vi "Recent History Buffer (Array(DBL)).vi"(8 "number of elements [init or read] (100)":i32=100, 9 "new element [write]":dbl format="%0.2f", 10 "mode [init:0;write:1;read:2]":enum16{"initialize", "write", "read"}(ring)) -> (1 "number to date":u32, 2 "requested elements [read]":dbl[](array[numeric]) format="%0.2f", 3 "buffer full?":bool)   [LabVIEW 2009]
doc: "This history buffer saves an internal 1D array of the most recent N values that it receives, where N is the number of elements specified when the buffer is initialized. \n\nThere are three modes to access this buffer - init, write, and read. You must first call the VI in init mode to set the buffer size. In write mode, each call writes a new element to the buffer, overwriting the oldest element if the buffer is full. In read mode, each call returns the lesser of the requested number of elements or the number currently stored in the buffer; element 0 is the oldest of the requested elements.\n\nSince this VI behaves like a global variable, it is called a \"functional global\". Search the LabVIEW Help for \"functional global\" for more information on the reasons you might use a functional global instead of a standard global variable."
panel:
  # "Press Ctrl-H for more information."
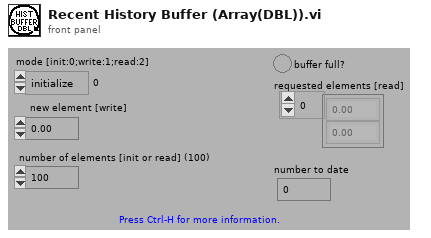
[diagram p1: front panel]
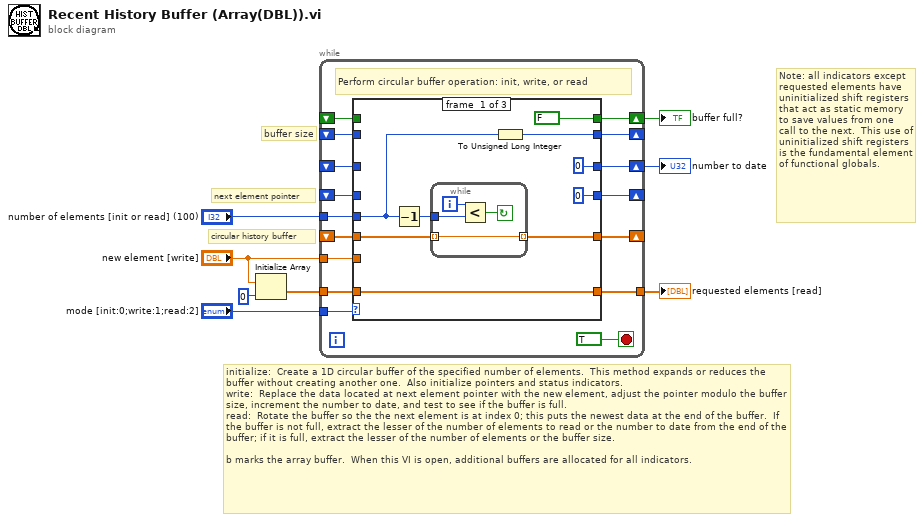
[diagram p0: block diagram]
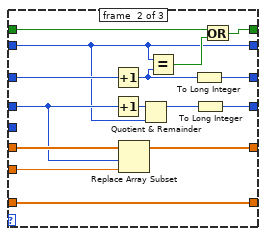
[diagram p2: hidden frame]
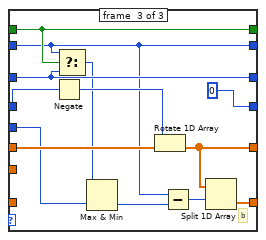
[diagram p3: hidden frame]
diagram:
  # "Note: all indicators except requested elements have uninitialized shift registers that act as static memory to save values from one call to the next.  This use of uninitialized shift registers is the fundamental element of functional globals."
  # "initialize:  Create a 1D circular buffer of the specified number of elements.  This method expands or reduces the buffer without creating another one.  Also initialize pointers and status indicators. \nwrite:  Replace the data located at next element pointer with the new element, adjust the pointer modulo the buffer size, increment the number to date, and test to see if the buffer is full.\nread:  Rotate the buffer so the the next element is at index 0; this puts the newest data at the end of the buffer.  If the buffer is not full, extract the lesser of the number of elements to read or the number to date from the end of the buffer; if it is full, extract the lesser of the number of elements or the buffer size.\n\nb marks the array buffer.  When this VI is open, additional buffers are allocated for all indicators."
  # "circular history buffer"
  # "next element pointer"
  # "buffer size"
  n1 = Initialize Array("new element [write]", 0) -> (w2:dbl[])
  n2 = while {
    tunnel: "mode [init:0;write:1;read:2]" -> [w24]
    tunnel: "number of elements [init or read] (100)" -> [w23]
    tunnel: "new element [write]" -> [w22]
    shift-right: [w21] -> w4
    shift-left: _ -> [w20]
    shift-right: [w17] -> _
    shift-left: _ -> [w18]
    shift-right: [w15] -> w3
    shift-left: _ -> [w16]
    shift-right: [w13] -> _
    shift-left: _ -> [w14]
    shift-right: [w11] -> _
    shift-left: _ -> [w12]
    tunnel: w2 -> [w10]
    tunnel: [w9] -> w1
    stop <- TRUE stop-if-true
    # "Perform circular buffer operation: init, write, or read"
    n3 = case "Perform circular buffer operation: init, write, or read" shown="\"initialize\"" w24 {
      tunnel: w18 -> [_ w39 w55]
      tunnel: [w25 w39 w55] -> w17
      tunnel: [w32 w48 w61] -> w9
      tunnel: w14 -> [_ w45 w54]
      tunnel: w22 -> [_ w41 _]
      tunnel: w12 -> [w30 w47 w64]
      tunnel: [0 w40 0] -> w13
      tunnel: [w29 w46 w63] -> w11
      tunnel: w23 -> [w28 _ w56]
      tunnel: [FALSE w49 w59] -> w21
      tunnel: w20 -> [_ w50 w59]
      tunnel: w10 -> [w32 w48 _]
      tunnel: [u32 0 w38 w58] -> w15
      tunnel: w16 -> [_ w44 w58]
      frame #0 {
        n4 = Decrement(x=w28) -> (x-1=w31:i32)
        n5 = while {
          tunnel: [w34] -> w29 mode=indexing
          tunnel: w30 -> [w34] mode=indexing
          tunnel: w31 -> [w37]
          i -> [w36]
          stop <- w35 continue-if-true
          n6 = Less?(x=w36, y=w37) -> (x < y?=w35:bool)
        }
        n7 = To Unsigned Long Integer(number=w28) -> (unsigned 32bit integer=w25:u32)
      }
      frame #1 {
        n8 = Increment(x=w44) -> (x+1=w42:u32)
        n9 = Increment(x=w45) -> (x+1=w51:i32)
        n10 = Replace Array Subset(array=w47, new element=w41, index=w45) -> (w46:dbl[])
        n11 = Quotient & Remainder(x=w51, y=w39) -> (x-y*floor(x/y)=w52:u32)  [unwired: 1 out]
        n12 = Equal?(x=w39, y=w42) -> (x = y?=w43:bool)
        n13 = To Long Integer(number=w42) -> (32bit integer=w38:i32)
        n14 = To Long Integer(number=w52) -> (32bit integer=w40:i32)
        n15 = Or(x=w50, y=w43) -> (x .or. y?=w49:bool)
      }
      frame #2 {
        # "b"
        n16 = Negate(x=w54) -> (-x=w65:i32)
        n17 = Select(t=w55, s=w59, f=w58) -> (s? t:f=w57:u32)
        n18 = Max & Min(x=w57, y=w56) -> (min(x,y)=w60:u32)  [unwired: 1 out]
        n19 = Rotate 1D Array(1:w64, 2:w65) -> (0:w63:dbl[])
        n20 = Subtract(x=w55, y=w60) -> (x-y=w53:u32)
        n21 = Split 1D Array(array=w63, index=w53) -> (second subarray=w61:dbl[])  [unwired: 1 out]
      }
    }
  }
  "requested elements [read]" <- w1
  "buffer full?" <- w4
  "number to date" <- w3
